vi "Classical Order Estimation Ripple Spec Cvt.vi"(10 "ripple specs":T1={"passband"=0.1, "stopband"=40.0, "dB/linear? (T: dB)"=TRUE}) -> (1 "ripple specs (dB)":T1={"passband"=0.0, "stopband"=0.0, "dB/linear? (T: dB)"=TRUE}, 2 "ripple specs (linear)":T1={"passband"=0.0, "stopband"=0.0, "dB/linear? (T: dB)"=TRUE})   [LabVIEW 2017, in "NI_AAL_Filter.lvlib"]
uses:
  <vilib>/Analysis/NI_AAL_Filter.lvlib
  <vilib>/Analysis/3filter.llb/Filter Ripple Specification (Design).ctl
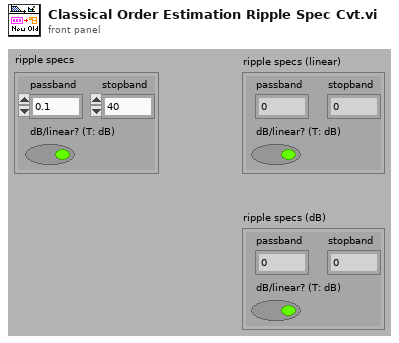
[diagram p1: front panel]
types:
  T1 = typedef "NI_AAL_Filter.lvlib/Filter Ripple Specification (Design).ctl" = cluster{"passband":dbl, "stopband":dbl, "dB/linear? (T: dB)":bool}
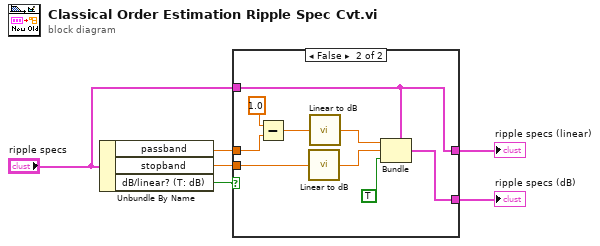
[diagram p0: block diagram]
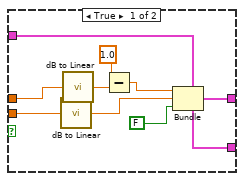
[diagram p2: hidden frame]
diagram:
  n1 = Unbundle By Name("ripple specs") -> ("passband"=w5:dbl, "stopband"=w4:dbl, "dB/linear? (T: dB)"=w6:bool)
  n2 = case shown="False" w6 {
    tunnel: w5 -> [w10 w22]
    tunnel: w4 -> [w8 w17]
    tunnel: [w12 w21] -> w2
    tunnel: "ripple specs" -> [w11 w21]
    tunnel: [w11 w20] -> w1
    frame True {
      n3 = call <vilib>:"dB to Linear.vi"("dB value"=w8) -> ("linear value"=w7:dbl)  [unwired: 1 in]
      n4 = call <vilib>:"dB to Linear.vi"("dB value"=w10) -> ("linear value"=w9:dbl)  [unwired: 1 in]
      n5 = Subtract(x=1.0, y=w9) -> (x-y=w14:dbl)
      n6 = Bundle(cluster=w11, "passband"=w14, "stopband"=w7, "dB/linear? (T: dB)"=FALSE ("dB/ripple level (T:dB)")) -> (w12:T1)
    }
    frame False {
      n7 = Subtract(x=1.0, y=w22) -> (x-y=w19:dbl)
      n8 = call <vilib>:"Linear to dB.vi"("linear value"=w17) -> ("dB value"=w16:dbl)  [unwired: 1 in]
      n9 = call <vilib>:"Linear to dB.vi"("linear value"=w19) -> ("dB value"=w18:dbl)  [unwired: 1 in]
      n10 = Bundle(cluster=w21, "passband"=w18, "stopband"=w16, "dB/linear? (T: dB)"=TRUE ("dB/ripple level (T:dB)")) -> (w20:T1)
    }
  }
  "ripple specs (linear)" <- w2
  "ripple specs (dB)" <- w1
